vi "compute Command Listener ID.vi"(0 "Listener Session ID":string, 2 "REx - Command ROOT":refnum<class "REx Command - Root.lvclass">, 11 "error in":errorcluster) -> (6 "Command Listener ID":string, 15 "error out":errorcluster)   [LabVIEW 2012, in "REx.lvlib" / "REx Command - Root.lvclass"]
uses:
  REx Command Root/REx Command - Root.lvclass
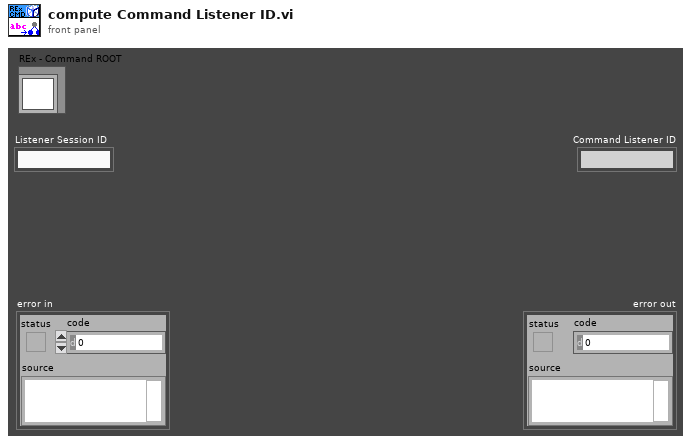
[diagram p1: front panel]
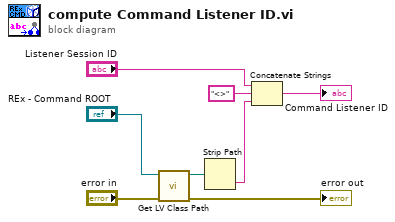
[diagram p0: block diagram]
diagram:
  n1 = call <vilib>:"Get LV Class Path.vi"("error in (no error)"="error in", "object"="REx - Command ROOT") -> ("error out"=→"error out":errorcluster, "class path"=w1:path)  [unwired: 8 in]
  n2 = Strip Path(path=w1) -> (name=w3:string)  [unwired: 1 out]
  n3 = Concatenate Strings("Listener Session ID", "<>" ("string"), w3) -> (→"Command Listener ID":string)
